vi "Process Flushed Data.vi"(8 "error in (no error)":errorcluster, 10 "Flushed Elements":T1[](array[typedef]), 11 "Report Generator in":refnum<class "Report Generator.lvclass">) -> (0 "error out":errorcluster, 3 "Report Generator out":refnum<class "Report Generator.lvclass">)   [LabVIEW 2023, in "Report Generator.lvlib" / "Report Generator.lvclass"]
doc: "This is the primary routine of the report generator dependant upn the logging enabled DVR\n\nIf logging is enabled this tool supports the following functions:\n<b>Open</b> This will open a new report \n<b>Close</b> This will close the report and remove report from memory\n<b>Multi-Chan</b> This will log multiple channel data to the provided group memory location\n<b>Event</b> This will log any event triggered by the software (defined to generate an event record)\n<b>Properties</b> This will assign properties to the provided group. If group is blank this will push the porperties to the test primary group."
uses:
  Library/Report Generator.lvclass
  C:/Users/Public/Documents/Development/builds/Framework/Engine.lvlibp/Engine/Library/Engine.lvclass
  builds/Tools/QDMH.lvlibp/Custom Controls/Message.ctl
  builds/Framework/Engine.lvlibp/Engine/Accessors/DVRs/Read Logging Enabled.vi
  builds/Framework/Engine.lvlibp/Engine/Library/Engine.lvclass
  builds/Tools/QDMH.lvlibp/Library/QDMH.lvclass
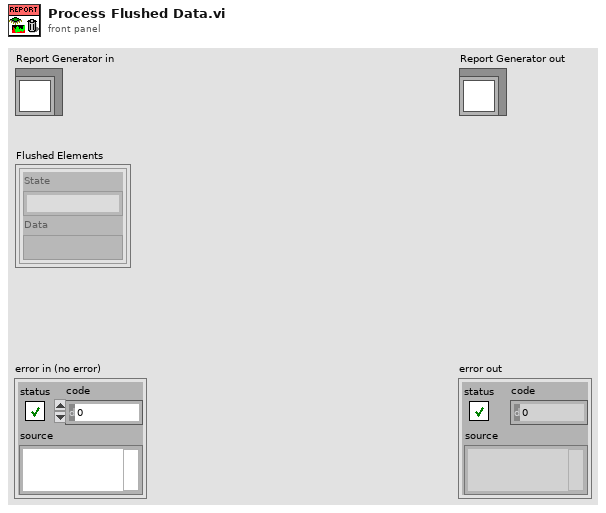
[diagram p1: front panel]
types:
  T1 = typedef "QDMH.lvlibp/QDMH.lvclass/Message.ctl" = cluster{"State":string, "Data":variant}
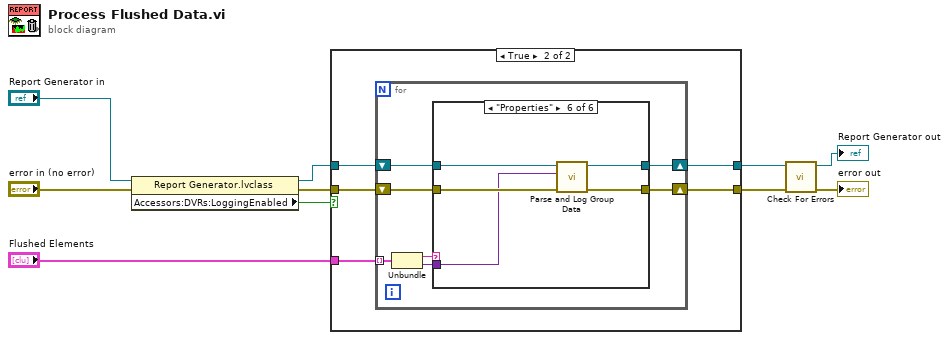
[diagram p0: block diagram]
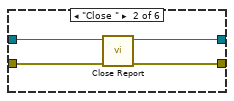
[diagram p4: hidden frame]
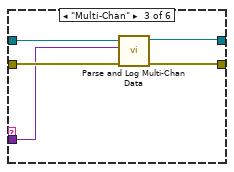
[diagram p5: hidden frame]
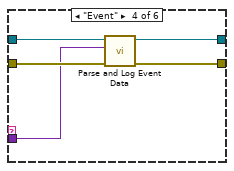
[diagram p6: hidden frame]
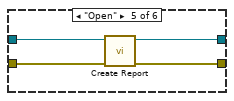
[diagram p7: hidden frame]
diagram:
  n1 = property class="Report Generator.lvclass"(reference="Report Generator in", error in="error in (no error)") -> (reference out=w2:refnum<class "Report Generator.lvclass">, error out=w4:errorcluster, "Accessors:DVRs:LoggingEnabled"=w1:bool)
  n2 = case shown="True" w1 {
    tunnel: "Flushed Elements" -> [_ w17]
    tunnel: w4 -> [w11 w16]
    tunnel: [w11 w15] -> w8
    tunnel: [w12 w14] -> w6
    tunnel: w2 -> [w12 w13]
    frame False {
    }
    frame True {
      n3 = for {
        tunnel: w17 -> [w24] mode=indexing
        shift-right: [w20] -> w15
        shift-left: w16 -> [w22]
        shift-right: [w21] -> w14
        shift-left: w13 -> [w19]
        n4 = Unbundle(w24) -> ("State"=w18:string, "Data"=w23:variant)
        n5 = case shown="\"Properties\"" w18 {
          tunnel: w19 -> [w26 w30 w33 w39 w44 w49]
          tunnel: [w26 w29 w32 w38 w43 w47] -> w21
          tunnel: w22 -> [w25 w28 w35 w40 w42 w48]
          tunnel: [w25 w27 w34 w37 w41 w46] -> w20
          tunnel: w23 -> [_ _ w31 w36 _ w45]
          frame Default {
          }
          frame "Close " {
            n6 = call-dynamic "Close Report.vi"("error in (no error)"=w28, "Report Generator in"=w30) -> ("error out"=w27:errorcluster, "Report Generator out"=w29:refnum<class "Report Generator.lvclass">)  [unwired: 8 in]
          }
          frame "Multi-Chan" {
            n7 = call "Parse and Log Multi-Chan Data.vi"("error in (no error)"=w35, "MultiChan Variant"=w31, "Report Generator in"=w33) -> ("error out"=w34:errorcluster, "Report Generator out"=w32:refnum<class "Report Generator.lvclass">)  [unwired: 7 in]
          }
          frame "Event" {
            n8 = call "Parse and Log Event Data.vi"("error in (no error)"=w40, "Event Variant"=w36, "Report Generator in"=w39) -> ("error out"=w37:errorcluster, "Report Generator out"=w38:refnum<class "Report Generator.lvclass">)  [unwired: 7 in]
          }
          frame "Open" {
            n9 = call "Create Report.vi"("error in (no error)"=w42, "Report Generator in"=w44) -> ("error out"=w41:errorcluster, "Report Generator out"=w43:refnum<class "Report Generator.lvclass">)  [unwired: 8 in]
          }
          frame "Properties" {
            n10 = call "Parse and Log Group Data.vi"("error in (no error)"=w48, "Data"=w45, "Report Generator in"=w49) -> ("error out"=w46:errorcluster, "Report Generator out"=w47:refnum<class "Report Generator.lvclass">)  [unwired: 7 in]
          }
        }
      }
    }
  }
  n11 = call "Check For Errors.vi"("error in"=w8, "Engine in"=w6) -> ("error out"=→"error out":errorcluster, "Engine out"=→"Report Generator out":refnum<class "Report Generator.lvclass">)  [unwired: 8 in]
